vi "Test Coffee Shop Added Customer Broadcasts Status.vi"(8 "error in (no error)":errorcluster, 11 "Coffee Shop Test In":refnum<class "Coffee Shop Test.lvclass">) -> (0 "error out":errorcluster, 3 "Coffee Shop Test Out":refnum<class "Coffee Shop Test.lvclass">)   [LabVIEW 2020, in "Coffee Shop Test.lvclass"]
uses:
  Coffee Shop Test.lvclass
  Coffee Shop/Coffee Shop.lvclass
  <vilib>/Asteme/Triarc Framework/Process/Process.lvclass
  <vilib>/Asteme/Triarc Framework/Application/Application.lvclass
  <vilib>/Asteme/Triarc Framework Test Suite/Support/Event Helpers/Event Helpers.lvlib
  C:/Program Files (x86)/National Instruments/LabVIEW 2020/vi.lib/Asteme/Triarc Framework/Application/Application.lvclass
  C:/Program Files (x86)/National Instruments/LabVIEW 2020/vi.lib/Asteme/Triarc Framework/Process/Process.lvclass
  C:/Program Files (x86)/National Instruments/LabVIEW 2020/vi.lib/Asteme/Triarc Framework/Base/Base.lvclass
  C:/Program Files (x86)/National Instruments/LabVIEW 2020/vi.lib/Asteme/Triarc Framework/Error Handler Interface/Error Handler Interface.lvclass
  C:/Program Files (x86)/National Instruments/LabVIEW 2020/vi.lib/Asteme/Triarc Framework/Logging/Logging.lvclass
  C:/Users/anton/Documents/GitHub/Triarc-Examples/Coffee Shop/Coffee Shop/Coffee Shop.lvclass
  <vilib>/Asteme/LUnit/Test Case.lvclass
  C:/Program Files (x86)/National Instruments/LabVIEW 2020/vi.lib/Asteme/Triarc Framework Test Suite/Application Test/Application Test.lvclass
  C:/Program Files (x86)/National Instruments/LabVIEW 2020/vi.lib/Asteme/Triarc Framework Test Suite/Process Test/Process Test.lvclass
  C:/Program Files (x86)/National Instruments/LabVIEW 2020/vi.lib/Asteme/Triarc Framework Test Suite/Base Class Test/Base Test.lvclass
  C:/Program Files (x86)/National Instruments/LabVIEW 2020/vi.lib/Asteme/LUnit/Test Case.lvclass
  C:/Users/anton/Documents/GitHub/Triarc-Examples/Coffee Shop/Coffee Shop Test/Coffee Shop Test.lvclass
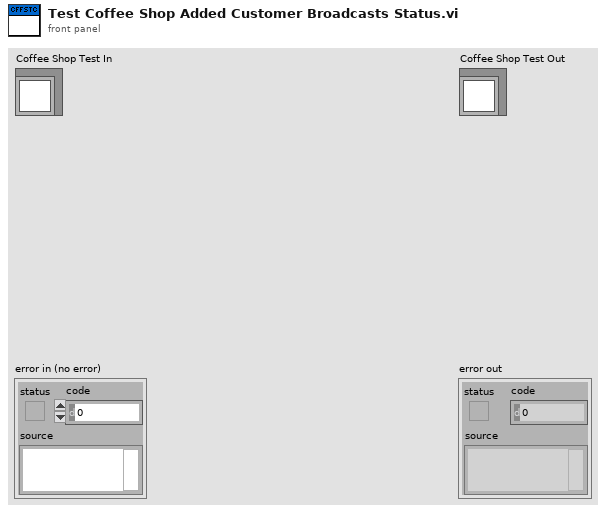
[diagram p1: front panel]
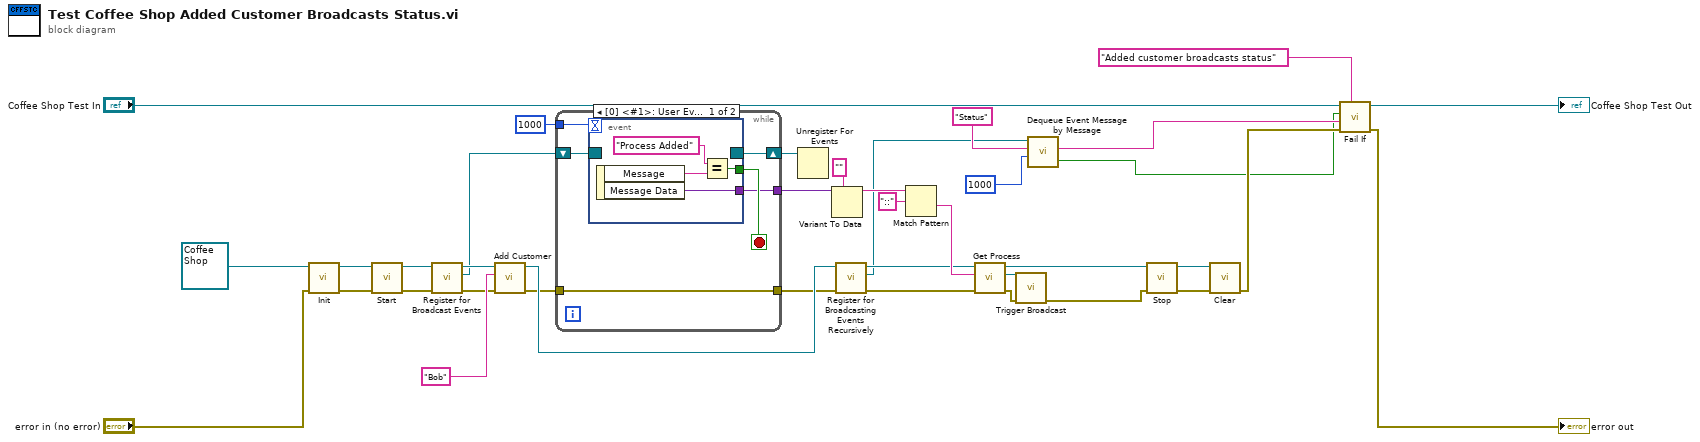
[diagram p0: block diagram]
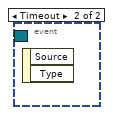
[diagram p2: hidden frame]
diagram:
  n1 = call-dynamic "Init.vi"("error in (no error)"="error in (no error)", "Process In"=refnum<class "Coffee Shop.lvclass"> refnum ("Coffee Shop.lvclass")) -> ("error out"=w36:errorcluster, "Process Out"=w37:refnum<class "Coffee Shop.lvclass">)  [unwired: 8 in]
  n2 = call <vilib>:"Start.vi"("error in (no error)"=w36, "Process In"=w37) -> ("error out"=w21:errorcluster, "Process Out"=w22:refnum<class "Coffee Shop.lvclass">)  [unwired: 8 in]
  n3 = call <vilib>:"Register for Broadcast Events.vi"("error in (no error)"=w21, "Process In"=w22) -> ("error out"=w19:errorcluster, "Event Registration Refnum Out"=w18:refnum<event-registration>, "Process Out"=w20:refnum<class "Coffee Shop.lvclass">)  [unwired: 7 in]
  n4 = call "Add Customer.vi"("error in (no error)"=w19, "Name"="Bob", "Coffee Shop in"=w20) -> ("error out"=w2:errorcluster, "Coffee Shop out"=w6:refnum<class "Coffee Shop.lvclass">)  [unwired: 7 in]
  n5 = while {
    shift-right: [w43] -> w17
    shift-left: w18 -> [w44]
    tunnel: 1000 -> [w42]
    tunnel: [w40] -> w15
    tunnel: [w39] -> w3
    tunnel: w2 -> [w39]
    stop <- w41 stop-if-true
    n6 = event shown="[0] <#1>: User Event" {
      selector: w44 -> [_ _]
      dyn-events: [_ _] -> w43
      timeout: w42 -> [_ _]
      tunnel: [w46 _] -> w41
      tunnel: [w45 _] -> w40
      event User Event {
        n7 = event-data() -> ("Message"=w48:string, "Message Data"=w45:variant)  [unwired: 1 in]
        n8 = Equal?(x="Process Added", y=w48) -> (x = y?=w46:bool)
      }
      event Timeout {
        n9 = event-data() -> ()  [unwired: 1 in, 2 out]
      }
    }
  }
  n10 = Unregister For Events(event registration refnum=w17) -> ()  [unwired: 1 in, 1 out]
  n11 = Variant To Data(type="", Variant=w15) -> (data=w12:string)  [unwired: 1 in, 1 out]
  n12 = call <vilib>:"Register for Broadcasting Events Recursively.vi"("error in (no error)"=w3, "Application In"=w6) -> ("error out"=w4:errorcluster, "Event Registration Refnum Out"=w1:refnum<event-registration>, "Application Out"=w5:refnum<class "Coffee Shop.lvclass">)  [unwired: 7 in]
  n13 = Match Pattern(string=w12, regular expression="::") -> (after substring=w9:string)  [unwired: 1 in, 3 out]
  n14 = call <vilib>:"Get Process.vi"("error in (no error)"=w4, "Process Name"=w9, "Rig In"=w5) -> ("error out"=w14:errorcluster, "App Process"=w7:refnum<class "Process.lvclass">, "Rig Out"=w13:refnum<class "Coffee Shop.lvclass">)  [unwired: 6 in]
  n15 = call <vilib>:"Trigger Broadcast.vi"("error in (no error)"=w14, "Process in"=w7) -> ("error out"=w8:errorcluster)  [unwired: 8 in, 1 out]
  n16 = call <vilib>:"Dequeue Event Message by Message.vi"("Timeout (-1)"=1000, "Message"="Status", "Event Registration Refnum"=w1) -> ("Message"=w24:string, "Timed Out?"=w23:bool)  [unwired: 4 in, 3 out]
  n17 = call <vilib>:"Stop.vi"("error in (no error)"=w8, "Process In"=w13) -> ("error out"=w34:errorcluster, "Process Out"=w35:refnum<class "Coffee Shop.lvclass">)  [unwired: 7 in, 1 out]
  n18 = call-dynamic "Clear.vi"("error in (no error)"=w34, "Application In"=w35) -> ("error out"=w30:errorcluster)  [unwired: 9 in]
  n19 = call <vilib>:"Fail If.vi"("Description"="Added customer broadcasts status", "error in (no error)"=w30, "Message"=w24, "Fail?"=w23, "Test Case In"="Coffee Shop Test In") -> ("error out"=→"error out":errorcluster, "Test Case Out"=→"Coffee Shop Test Out":refnum<class "Coffee Shop Test.lvclass">)  [unwired: 5 in]
